vi "Build.vi"(6 "Version":T2, 7 "Build Events":refnum<class "Build Events API.lvclass">, 8 "error in (no error)":errorcluster, 10 "Build Info":T1, 11 "Build in":refnum<class "Build.lvclass">) -> (0 "error out":errorcluster)   [LabVIEW 2020, in "Builder Tools.lvlib" / "Build.lvclass"]
uses:
  Build.lvclass
  Builder Core/Version.ctl
  Builder Core/Builder Core.lvlib
  Build Events API/Build Events API.lvclass
  Build Info.ctl
  Builder Tools.lvlib
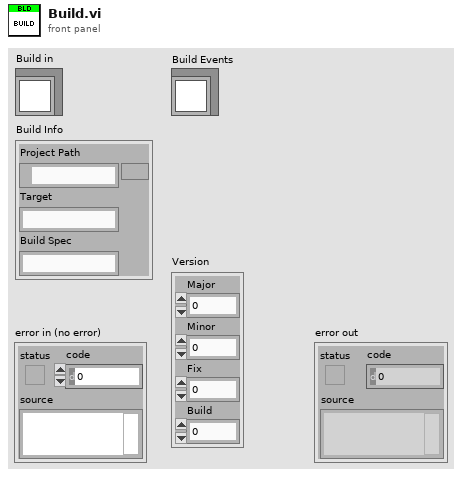
[diagram p1: front panel]
types:
  T1 = typedef "Builder Tools.lvlib/Build Info.ctl" = cluster{"Project Path":path, "Target":string, "Build Spec":string}
  T2 = typedef "Builder Core.lvlib/Version.ctl" = cluster{"Major":u16, "Minor":u16, "Fix":u16, "Build":u16}
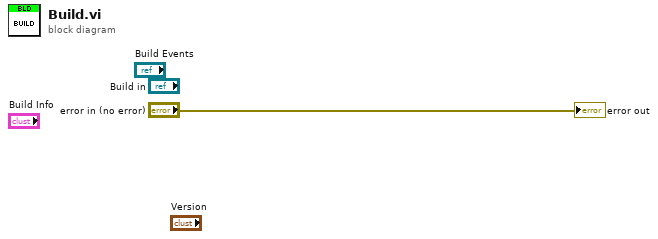
[diagram p0: block diagram]
diagram:
  "error out" <- "error in (no error)"
